vi "ManualControlL0.vi"() -> ()   [LabVIEW 2012]
uses:
  <vilib>/Utility/NIReport.llb/NI_report.lvclass
  <vilib>/Utility/NIReport.llb/HTML/NI_HTML.lvclass
  <instrlib>/Agilent 8000 Series/Public/Configure/Configure Math (Binary Operation).vi
  <instrlib>/Agilent 8000 Series/Agilent 8000 Series.lvlib
panel:
  in  "Control\nGenNOsc":bool=TRUE
  in  "IPR?":bool=TRUE
  out "Data":string="empty_read_buffer0_2-65@1\r\n0_2-70@0\r\n"
  out "IPR_count":u32
  in  "Sum/Maj 2":bool=TRUE
  in  "Treshold":i16=577 min=0 max=1000
  in  "Gen Active":bool=TRUE
  in  "Amp Scaler":dbl(slide)=2.519968045974613 scale=0.1..125.0
  in  "Voltage Input":dbl(slide)=0.5025139664804469 scale=0.05..0.8
  in  "Sum/Maj":bool=TRUE
  in  "Ib Clip select":i32(slide)=63 scale=0.0..63.0
  in  "Clipping Select":i32(slide)=1 scale=1.0..3.0
  in  "Attenuation Select":i32(slide) scale=0.0..15.0
  in  "Delay Enable":i32
  in  "Channel Enable":i32(slide) scale=0.0..6.0
  in  "stop":bool
  in  "Instrument VISA in":T1={"AWG VISA"="AgilentGen1", "Oscilloscope  VISA "="AgilentOsc", "Integration Board IP"="172.16.17.47", "connection ID"=refnum, "report out"=refnum, "report file path"=path "C:/Users/omartinez/Desktop/L0nL1_Results"}
  out "error out":errorcluster
  in  "error in":errorcluster
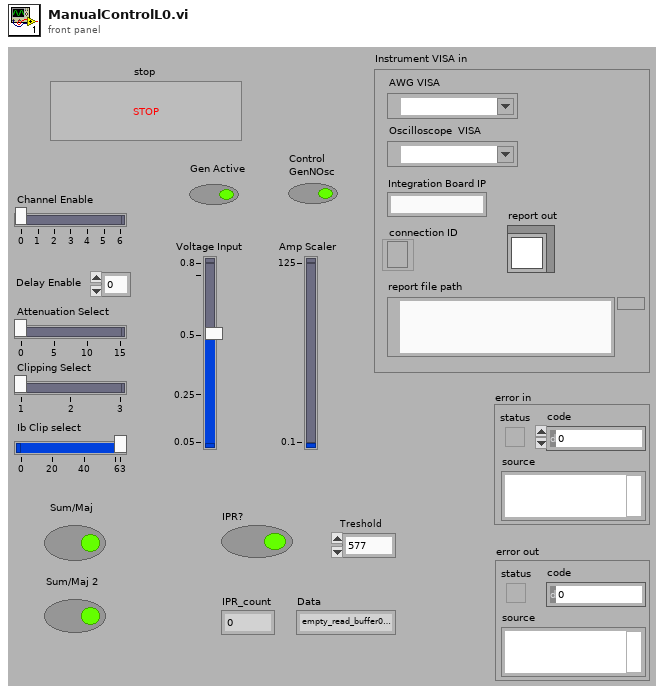
[diagram p1: front panel]
types:
  T1 = cluster{"AWG VISA":refnum<visa-resource-name>, "Oscilloscope  VISA ":refnum<visa-resource-name>, "Integration Board IP":string, "connection ID":refnum<k5>, "report out":refnum<class "NI_report.lvclass">, "report file path":path}
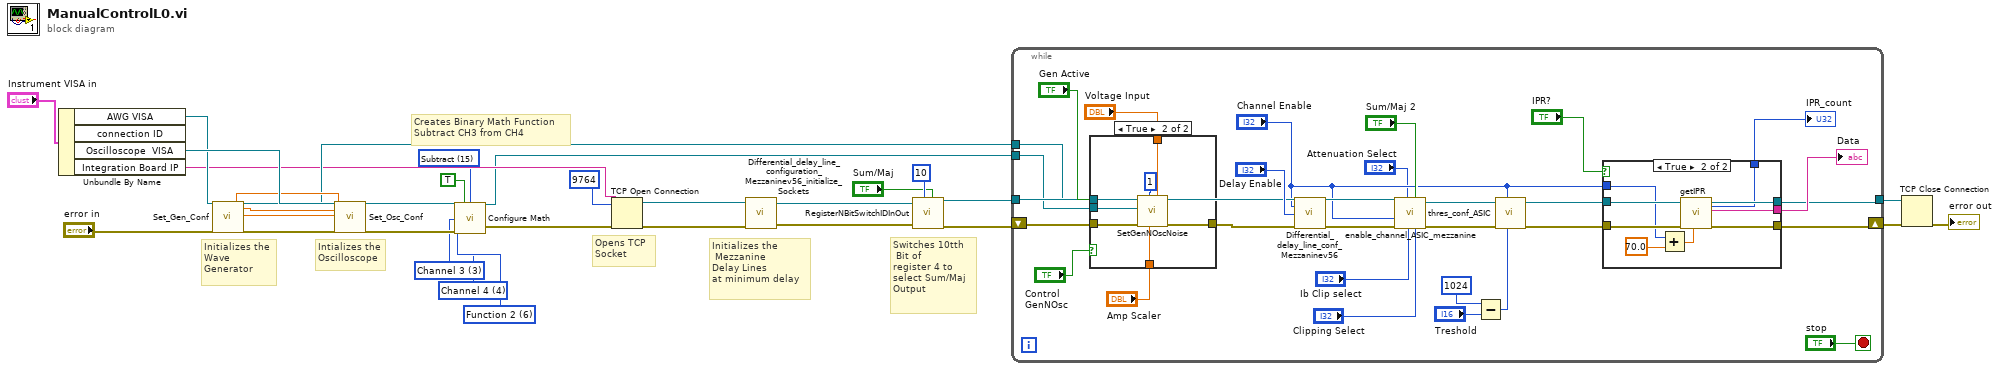
[diagram p0: block diagram]
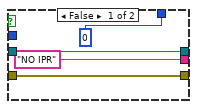
[diagram p3: hidden frame]
diagram:
  w16 = u16 6 items=["Function 1"=5, "Function 2"=6, "Function 3"=7, "Function 4"=8] ("Math Channel (5: Function 1)")
  w17 = u16 15 items=["Add"=12, "Divide"=13, "Multiply"=14, "Subtract"=15, "Common Mode"=16, "Versus"=17] ("Math Operation (12: Add)")
  w11 = 3 items=["Channel 1"=1, "Channel 2"=2, "Channel 3"=3, "Channel 4"=4] ("Channel (1: Channel 1)")
  w12 = 4 items=["Channel 1"=1, "Channel 2"=2, "Channel 3"=3, "Channel 4"=4] ("Channel (1: Channel 1)")
  # "Initializes the\n Mezzanine\nDelay Lines \nat minimum delay"
  # "Switches 10tth \n Bit of\nregister 4 to \nselect Sum/Maj\nOutput"
  # "Opens TCP\nSocket"
  # "Creates Binary Math Function\nSubtract CH3 from CH4"
  # "Intializes the\nOscilloscope"
  # "Initializes the \nWave\nGenerator"
  n1 = Unbundle By Name("Instrument VISA in") -> ("AWG VISA"=w26:refnum<visa-resource-name>, "Oscilloscope  VISA"=w27:refnum<visa-resource-name>, "Integration Board IP"=w19:string)  [unwired: 1 out]
  n2 = call "Set_Gen_Conf.vi"("AWG VISA"=w26, "error in (no error)"="error in") -> ("Amplitude 1 OUT"=w24:dbl, "VISA resource name out"=w20:refnum<visa-resource-name>, "Pulse Width in seconds 1 OUT"=w23:dbl, "Trigger Level 1"=w22:dbl, "error out"=w29:errorcluster)  [unwired: 10 in, 3 out]
  n3 = call "Set_Osc_Conf.vi"("VISA resource name"=w27, "Amplitude IN"=w24, "Trigger Level IN"=w22, "Pulse Width in seconds IN"=w23, "error in (no error)"=w29) -> ("VISA resource name out"=w15:refnum<visa-resource-name>, "error out"=w13:errorcluster)  [unwired: 13 in]
  n4 = call-poly <instrlib>:"Configure Math.vi"("VISA resource name"=w15, "Enable Math Channel (T:Enable)"=TRUE, "Math Operation (12: Add)"=w17, "Math Channel (5: Function 1)"=w16, "Math Operand (1: Channel 1)"=w11, "Math Operand (2: Channel 2)"=w12, "error in (no error)"=w13) -> ("VISA resource name out"=w14:refnum<visa-resource-name>, "error out"=w5:errorcluster)  [unwired: 7 in]
  n5 = TCP Open Connection(address=w19, remote port or service name=9764, error in (no error)=w5) -> (connection ID=w2:refnum<k5>, error out=w4:errorcluster)  [unwired: 2 in]
  n6 = call "Differential_delay_line_configuration_Mezzaninev56_initialize_Sockets.vi"("connection ID"=w2, "error in (no error)"=w4) -> ("connection ID out"=w1:refnum<k5>, "error out 2"=w3:errorcluster)  [unwired: 6 in]
  n7 = call "RegisterNBitSwitchIDInOut.vi"("Switch Bit"="Sum/Maj", "N Bit"=10, "error in (no error)"=w3, "connection ID"=w1) -> ("error out"=w9:errorcluster, "connection ID out"=w8:refnum<k5>)  [unwired: 5 in]
  n8 = while {
    tunnel: w14 -> [w49]
    tunnel: w20 -> [w48]
    tunnel: w8 -> [w50]
    tunnel: [w40] -> w6
    shift-right: [w39] -> w21
    shift-left: w9 -> [w47]
    stop <- "stop" stop-if-true
    n9 = case shown="True" "Control\nGenNOsc" {
      tunnel: [w62 w70] -> w61
      tunnel: "Voltage Input" -> [_ w69]
      tunnel: "Amp Scaler" -> [_ w68]
      tunnel: "Gen Active" -> [_ w67]
      tunnel: w49 -> [_ w66]
      tunnel: w48 -> [_ w65]
      tunnel: w47 -> [w62 w64]
      frame False {
      }
      frame True {
        n10 = call "SetGenNOscNoise.vi"("Enable Output"=w67, "Input Voltage"=w69, "Amp Scaler"=w68, "NChannels"=1, "error in (no error)"=w64, "Oscilloscope VISA"=w66, "Generator VISA"=w65) -> ("error out 2"=w70:errorcluster)  [unwired: 4 in]
      }
    }
    n11 = call "Differential_delay_line_conf_Mezzaninev56.vi"("connection ID"=w50, "channel"="Channel Enable", "Delay value"="Delay Enable", "error in (no error)"=w61) -> ("connection ID out"=w57:refnum<k5>, "error out 2"=w58:errorcluster)  [unwired: 4 in, 6 out]
    n12 = call "enable_channel_ASIC_mezzanine.vi"("Clip_sel_b"="Clipping Select", "maj/sum"="Sum/Maj 2", "Ib_clipVb"="Ib Clip select", "Att gain"="Attenuation Select", "error in"=w58, "Channel"="Channel Enable", "connection ID"=w57) -> ("error out"=w37:errorcluster, "connection ID out"=w36:refnum<k5>)  [unwired: 2 in, 1 out]
    n13 = Subtract(x=i16 1024, y="Treshold") -> (x-y=w34:i16)
    n14 = call "thres_conf_ASIC.vi"("threshold"=w34, "Ring"="Channel Enable", "error out 3"=w37, "connection ID"=w36) -> ("error out 2"=w35:errorcluster, "connection ID out"=w42:refnum<k5>)  [unwired: 4 in, 2 out]
    n15 = case shown="True" "IPR?" {
      tunnel: w35 -> [w74 w83]
      tunnel: [w74 w75] -> w39
      tunnel: w42 -> [w73 w82]
      tunnel: [w73 w81] -> w40
      tunnel: [u32 0 ("IPR_count") w78] -> w45
      tunnel: ["NO IPR" ("Data") w77] -> w44
      tunnel: "Channel Enable" -> [_ w76]
      frame False {
      }
      frame True {
        n16 = Add(x=w76, y=70.0) -> (x+y=w80:dbl)
        n17 = call "getIPR.vi"("Address"=w80, "error in"=w83, "connection ID"=w82) -> ("error out"=w75:errorcluster, "Data"=w77:string, "connection ID out"=w81:refnum<k5>, "IPR_count"=w78:u32)  [unwired: 5 in]
      }
    }
    "IPR_count" <- w45
    "Data" <- w44
  }
  n18 = TCP Close Connection(connection ID=w6, error in (no error)=w21) -> (error out=→"error out":errorcluster)  [unwired: 1 in, 1 out]
